vi "Initialize.vi"(7 "Serial Configuration":T1={"Baud Rate"=9600, "Parity"=0, "Data Bits"=8, "Stop Bits"=10} {"Stop Bits" items=["1.0"=10, "1.5"=15, "2.0"=20]; "Data Bits" items=["7"=7, "8"=8]; "Parity" items=["None", "Odd", "Even", "Mark", "Space"]; "Baud Rate" items=["300"=300, "600"=600, "1200"=1200, "2400"=2400, "4800"=4800, "9600"=9600, "19200"=19200]}, 8 "error in":errorcluster, 9 "Reset":bool=TRUE, 10 "ID Query":bool=TRUE, 11 "VISA resource name":refnum<visa-resource-name>) -> (0 "error out":errorcluster, 3 "VISA resource name out":refnum<visa-resource-name>)   [LabVIEW 2018, in "IT-M3100.lvlib"]
doc: "Establishes communication with the instrument and optionally performs an instrument identification query and/or an instrument reset. It also places the instrument in a default state needed for other instrument driver operations. Therefore, call this VI before calling other instrument driver VIs for this instrument. Generally, you need to call the <b>Initialize</b> VI only once at the beginning of an application."
uses:
  IT-M3100.lvlib
panel:
  # "(c) 2014 <Enter Company Name Here>.  ALL RIGHTS RESERVED."
  # "EDIT: Change control description to remove example text for buses not supported."
  # "EDIT: Serial settings must match those on the physical instrument.  Review user's manual to determine the correct Flow Control protocol for the instrument.  \"None\" is the least robust option for this setting, and could lead to unreliable data transmission."
  # "EDIT: If your instrument does not support ID query or Reset, remove the ID Query or Reset control from the front panel and delete the case structure with the ID Query or Reset code from the block diagram."
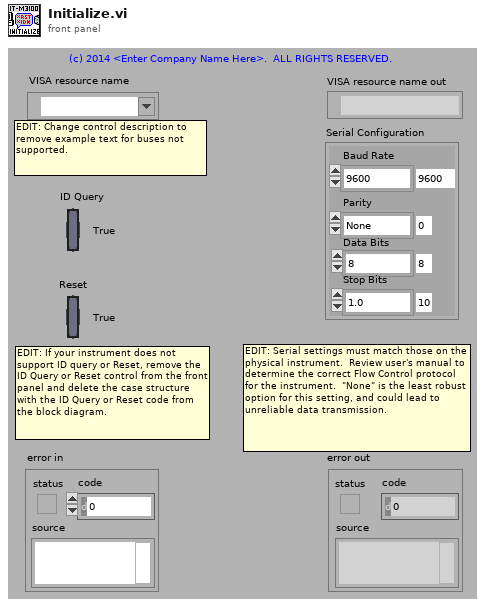
[diagram p1: front panel]
types:
  T1 = cluster{"Baud Rate":u32, "Parity":u16, "Data Bits":u16, "Stop Bits":u16}
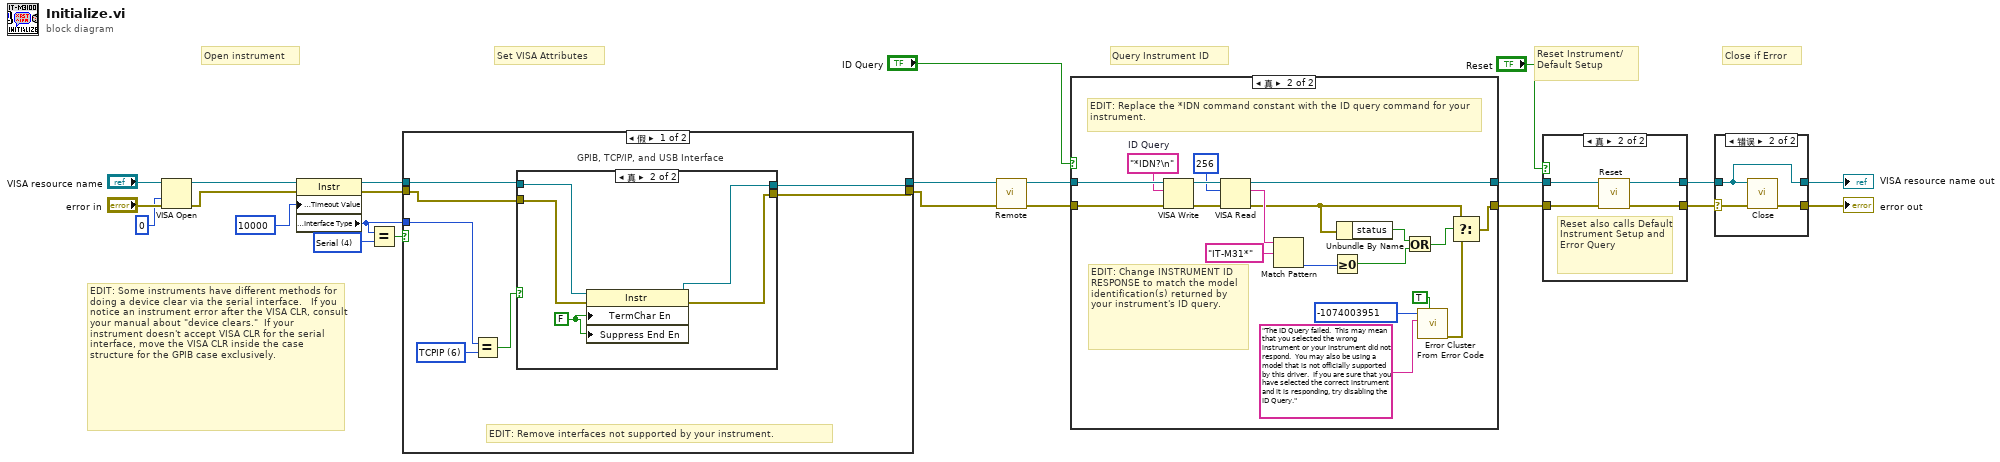
[diagram p0: block diagram]
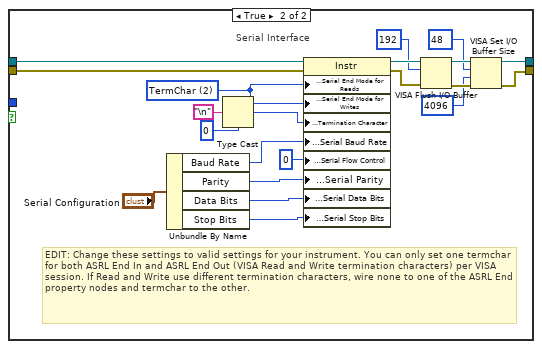
[diagram p3: hidden frame]
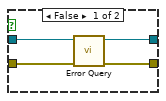
[diagram p5: hidden frame]
diagram:
  w13 = u16 4 items=["GPIB"=1, "VXI"=2, "GPIB-VXI"=3, "Serial"=4, "PXI"=5, "TCPIP"=6, "USB"=7] ("Interface Information:Interface Type")
  # "EDIT: Some instruments have different methods for doing a device clear via the serial interface.   If you notice an instrument error after the VISA CLR, consult your manual about \"device clears.\"  If your instrument doesn't accept VISA CLR for the serial interface, move the VISA CLR inside the case  structure for the GPIB case exclusively."
  # "Set VISA Attributes"
  # "Close if Error"
  # "Query Instrument ID"
  # "Reset Instrument/\nDefault Setup"
  # "Open instrument"
  n1 = VISA Open(access mode=u32 0, error in (no error)="error in", VISA resource name="VISA resource name") -> (VISA resource name=w11:refnum<visa-resource-name>, error out=w10:errorcluster)  [unwired: 2 in]
  n2 = property class="Instr"(reference=w11, error in=w10, "General Settings:Timeout Value"=u32 10000) -> (reference out=w16:refnum<visa-resource-name>, error out=w15:errorcluster, "Interface Information:Interface Type"=w1:u16)
  n3 = Equal?(x=w1, y=w13) -> (x = y?=w14:bool)
  n4 = case shown="假" w14 {
    tunnel: [w28 w55] -> w3
    tunnel: [w27 w52] -> w2
    tunnel: w16 -> [w30 w57]
    tunnel: w15 -> [w29 w58]
    tunnel: w1 -> [w24 _]
    frame False {
      w26 = u16 6 items=["GPIB"=1, "VXI"=2, "GPIB-VXI"=3, "Serial"=4, "PXI"=5, "TCPIP"=6, "USB"=7] ("Interface Information:Interface Type")
      # "EDIT: Remove interfaces not supported by your instrument."
      # "GPIB, TCP/IP, and USB Interface"
      n5 = Equal?(x=w24, y=w26) -> (x = y?=w25:bool)
      n6 = case shown="真" w25 {
        tunnel: [w32 w37] -> w28
        tunnel: [w31 w36] -> w27
        tunnel: w30 -> [w32 w35]
        tunnel: w29 -> [w31 w34]
        frame False {
        }
        frame True {
          w33 = FALSE
          n7 = property class="Instr"(reference=w35, error in=w34, "TermChar En"=w33, "Suppress End En"=w33) -> (reference out=w37:refnum<visa-resource-name>, error out=w36:errorcluster)
        }
      }
    }
    frame True {
      w45 = u16 2 items=["None", "LastBit", "TermChar"] ("Serial Settings:Serial End Mode for Reads")
      # "EDIT: Change these settings to valid settings for your instrument. You can only set one termchar for both ASRL End In and ASRL End Out (VISA Read and Write termination characters) per VISA session. If Read and Write use different termination characters, wire none to one of the ASRL End property nodes and termchar to the other."
      # "Serial Interface"
      n8 = Unbundle By Name("Serial Configuration") -> ("Baud Rate"=w43:u32, "Parity"=w41:u16, "Data Bits"=w42:u16, "Stop Bits"=w39:u16)
      n9 = Type Cast(type=u8 0, x="\n" ("Line Feed Constant")) -> (*(type *) &x=w44:u8)
      n10 = property class="Instr"(reference=w57, error in=w58, "Serial Settings:Serial End Mode for Reads"=w45, "Serial Settings:Serial End Mode for Writes"=w45, "Message Based Settings:Termination Character"=w44, "Serial Settings:Serial Baud Rate"=w43, "Serial Settings:Serial Flow Control"=0, "Serial Settings:Serial Parity"=w41, "Serial Settings:Serial Data Bits"=w42, "Serial Settings:Serial Stop Bits"=w39) -> (reference out=w51:refnum<visa-resource-name>, error out=w54:errorcluster)
      n11 = VISA Flush I/O Buffer(VISA resource name=w51, mask (16)=u16 192, error in (no error)=w54) -> (VISA resource name out=w56:refnum<visa-resource-name>, error out=w53:errorcluster)
      n12 = VISA Set I/O Buffer Size(VISA resource name=w56, mask (16)=u16 48, size (4096)=u32 4096 ("size (0)"), error in (no error)=w53) -> (VISA resource name out=w55:refnum<visa-resource-name>, error out=w52:errorcluster)
    }
  }
  n13 = call "Remote.vi"("error in"=w2, "VISA resource name"=w3) -> ("error out"=w4:errorcluster, "VISA resource name out"=w5:refnum<visa-resource-name>)  [unwired: 8 in]
  n14 = case shown="真" "ID Query" {
    tunnel: [w59 w79] -> w22
    tunnel: [w60 w76] -> w23
    tunnel: w5 -> [w60 w77]
    tunnel: w4 -> [w59 w78]
    frame False {
    }
    frame True {
      w70 = "*IDN?\n"  # ID Query
      # "EDIT: Replace the *IDN command constant with the ID query command for your instrument."
      # "EDIT: Change INSTRUMENT ID RESPONSE to match the model identification(s) returned by your instrument's ID query."
      n15 = VISA Write(VISA resource name=w77, write buffer=w70, error in (no error)=w78) -> (VISA resource name out=w74:refnum<visa-resource-name>, error out=w73:errorcluster)  [unwired: 1 out]
      n16 = VISA Read(VISA resource name=w74, byte count=u32 256, error in (no error)=w73) -> (VISA resource name out=w76:refnum<visa-resource-name>, read buffer=w75:string, error out=w64:errorcluster)  [unwired: 1 out]
      n17 = Match Pattern(string=w75, regular expression="IT-M31*") -> (offset past match=w65:i32)  [unwired: 1 in, 3 out]
      n18 = Greater Or Equal To 0?(x=w65) -> (x >= 0?=w62:bool)
      n19 = Unbundle By Name(w64) -> ("status"=w63:bool)
      n20 = Or(x=w63, y=w62) -> (x .or. y?=w61:bool)
      n21 = call <vilib>:"Error Cluster From Error Code.vi"("show call chain? (False)"=TRUE, "error message (\"\")"="The ID Query failed.  This may mean that you selected the wrong instrument or your instrument did not respond.  You may also be using a model that is not officially supported by this driver.  If you are sure that you have selected the correct instrument and it is responding, try disabling the ID Query." ("Source (VI Name)"), "error code (0)"=-1074003951 ("Code")) -> ("error out"=w69:errorcluster)  [unwired: 6 in]
      n22 = Select(t=w64, s=w61, f=w69) -> (s? t:f=w79:errorcluster)
    }
  }
  n23 = case shown="真" "Reset" {
    tunnel: w22 -> [w82 w84]
    tunnel: [w80 w87] -> w6
    tunnel: w23 -> [w83 w85]
    tunnel: [w81 w86] -> w7
    frame False {
      n24 = call "Error Query.vi"("error in"=w82, "VISA resource name"=w83) -> ("error out"=w80:errorcluster, "VISA resource name out"=w81:refnum<visa-resource-name>)  [unwired: 6 in, 2 out]
    }
    frame True {
      # "Reset also calls Default Instrument Setup and Error Query"
      n25 = call "Reset.vi"("error in"=w84, "VISA resource name"=w85) -> ("error out"=w87:errorcluster, "VISA resource name out"=w86:refnum<visa-resource-name>)  [unwired: 8 in]
    }
  }
  n26 = case shown="错误" w6 {
    selector: w6 -> [w88 w91]
    tunnel: w7 -> [w89 w90]
    tunnel: [w89 w90] -> w9
    tunnel: [w88 w92] -> w8
    frame No Error {
    }
    frame Error {
      n27 = call "Close.vi"("error in"=w91, "VISA resource name"=w90) -> ("error out"=w92:errorcluster)  [unwired: 9 in]
    }
  }
  "VISA resource name out" <- w9
  "error out" <- w8
